vi "Convert SAP CTCL Report File to Table.vi"(0 "File Path":path=path "C:/Users/rgenaway/Documents/Singapore Schedule Control/Workcenter Reports/CTCLActivitySing.txt", 1 "Sing Time Zone":bool) -> (7 "Converted Data Table":string[][](table), 8 "last mod":u32 format="%<%I:%M:%S %p\n%m/%d/%Y>T")   [LabVIEW 2018]
uses:
  <vilib>/Utility/file.llb/Read Delimited Spreadsheet (string).vi
panel:
  out "Start Index":i32
  out "all rows":string[][](array[string])
  # "This VI is used to convert a SAP text file into a Labview Table."
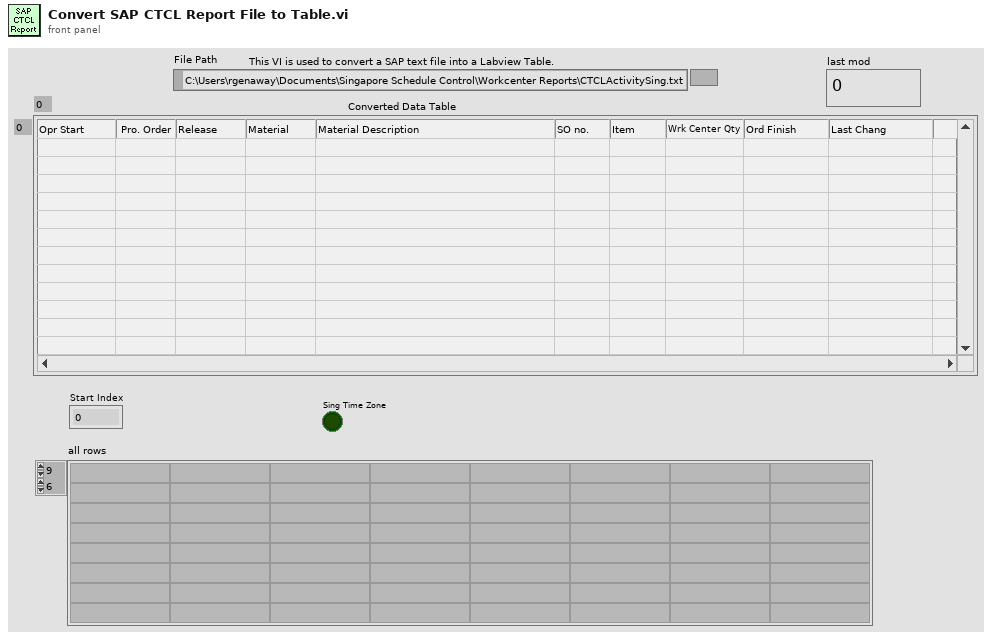
[diagram p1: front panel]
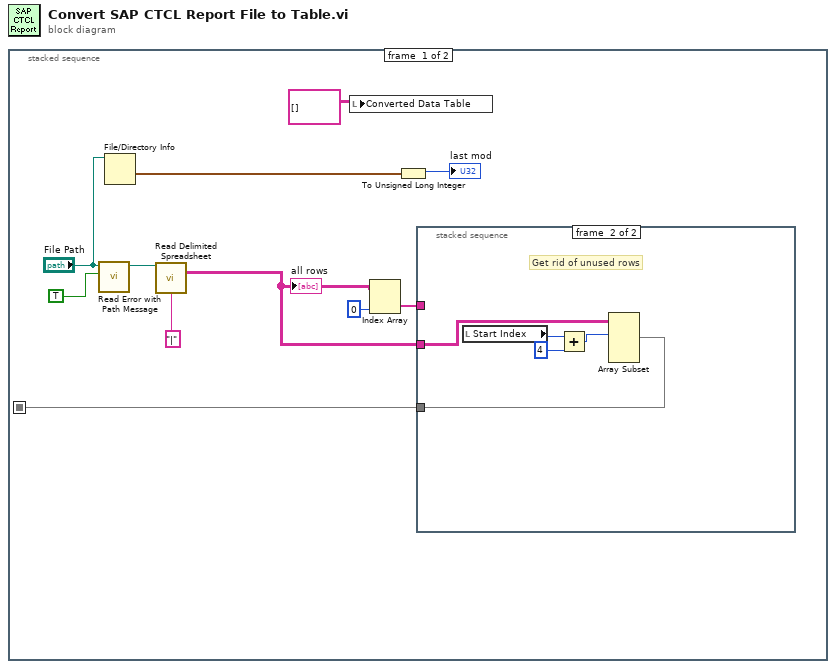
[diagram p0: block diagram]
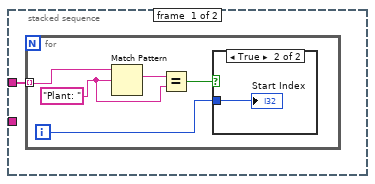
[diagram p2: hidden frame]
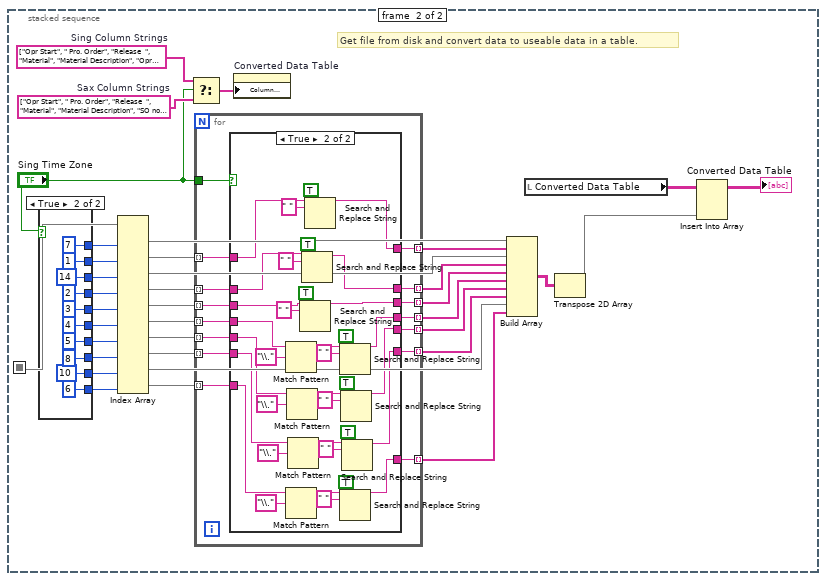
[diagram p4: hidden frame]
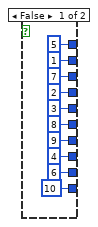
[diagram p5: hidden frame]
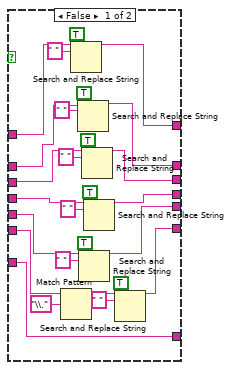
[diagram p6: hidden frame]
diagram:
  n1 = stacked-sequence {
    seq-local: [w8 _] -> [_ w46]
    frame #0 {
      n2 = call "Read Error with Path Message.vi"("quit? (T)"=TRUE, "Path"="File Path") -> ("path out"=w3:path)  [unwired: 8 in, 1 out]
      n3 = File/Directory Info(path="File Path") -> (last mod=w11:timestamp)  [unwired: 1 in, 6 out]
      n4 = call-poly <vilib>:"Read Delimited Spreadsheet.vi"("file path (dialog if empty)"=w3, "delimiter (\\t)"="|" ("delimiter (\\t)")) -> ("all rows"=w1:string[][])  [unwired: 8 in, 5 out]
      "all rows" <- w1
      n5 = local write "Converted Data Table"(string[][] [] ("Table")) -> ()
      n6 = Index Array(array=w1, index (col)=0 ("disabled index (col)")) -> (element=w5:string[])  [unwired: 1 in]
      n7 = To Unsigned Long Integer(number=w11) -> (unsigned 32bit integer=→"last mod":u32)
      n8 = stacked-sequence {
        tunnel: w5 -> [w12 _]
        tunnel: w1 -> [_ w23]
        tunnel: [_ w22] -> w8
        frame #0 {
          n9 = for {
            tunnel: w12 -> [w17] mode=indexing
            i -> [w13]
            w15 = "Plant: "
            n10 = Match Pattern(string=w17, regular expression=w15) -> (match substring=w16:string)  [unwired: 1 in, 3 out]
            n11 = Equal?(x=w16, y=w15) -> (x = y?=w14:bool)
            n12 = case shown="True" w14 {
              tunnel: w13 -> [_ w18]
              frame False {
              }
              frame True {
                "Start Index" <- w18
              }
            }
          }
        }
        frame #1 {
          # "Get rid of unused rows"
          n13 = local read "Start Index"() -> (w21:i32)
          n14 = Add(x=w21, y=4) -> (x+y=w19:i32)
          n15 = Array Subset(array=w23, index (row)=w19) -> (w22:string[][])  [unwired: 3 in]
        }
      }
    }
    frame #1 {
      w30 = string[] ["Opr Start", " Pro. Order", "Release  ", "Material", "Material Description", "Opr Qty", "Conf. Qty", "Wrk Center Qty", "Ord Finish", "Open Qty"]  # Sing Column Strings
      w29 = string[] ["Opr Start", " Pro. Order", "Release  ", "Material", "Material Description", "SO no.", "Item", "Wrk Center Qty", "Ord Finish", "Last Chang"]  # Sax Column Strings
      # "Get file from disk and convert data to useable data in a table."
      n16 = case shown="True" "Sing Time Zone" {
        tunnel: [5 ("disabled index (col)") 7 ("disabled index (col)")] -> w56
        tunnel: [1 ("index (col)") 1 ("index (col)")] -> w55
        tunnel: [7 ("index (col)") 14 ("index (col)")] -> w54
        tunnel: [2 ("index (col)") 2 ("index (col)")] -> w53
        tunnel: [3 ("index (col)") 3 ("index (col)")] -> w52
        tunnel: [8 ("index (col)") 4 ("index (col)")] -> w51
        tunnel: [9 ("index (col)") 5 ("index (col)")] -> w50
        tunnel: [4 ("index (col)") 8 ("index (col)")] -> w49
        tunnel: [6 ("index (col)") 10 ("index (col)")] -> w48
        tunnel: [10 ("index (col)") 6 ("index (col)")] -> w45
        frame False {
        }
        frame True {
        }
      }
      n17 = Index Array(array=w46, index (col) #1=w56, index (col) #2=w55, index (col) #3=w54, index (col) #4=w53, index (col) #5=w52, index (col) #6=w51, index (col) #7=w50, index (col) #8=w49, index (col) #9=w48, index (col) #10=w45) -> (element #1=w42:string[], element #2=w41:string[], element #3=w39:string[], element #4=w38:string[], element #5=w27:string[], element #6=w36:string[], element #7=w34:string[], element #8=w44:string[], element #9=w32:string[], element #10=w25:string[])  [unwired: 10 in]
      n18 = Select(t=w30, s="Sing Time Zone", f=w29) -> (s? t:f=w31:string[])
      n19 = for {
        tunnel: w44 -> [w94] mode=indexing
        tunnel: [w85] -> w43 mode=indexing
        tunnel: w41 -> [w93] mode=indexing
        tunnel: [w92] -> w40 mode=indexing
        tunnel: w38 -> [w91] mode=indexing
        tunnel: [w90] -> w37 mode=indexing
        tunnel: w36 -> [w89] mode=indexing
        tunnel: [w88] -> w35 mode=indexing
        tunnel: w34 -> [w87] mode=indexing
        tunnel: [w86] -> w33 mode=indexing
        tunnel: "Sing Time Zone" -> [w84]
        tunnel: w27 -> [w83] mode=indexing
        tunnel: [w82] -> w26 mode=indexing
        tunnel: w25 -> [w81] mode=indexing
        tunnel: [w80] -> w24 mode=indexing
        n20 = case shown="True" w84 {
          tunnel: w94 -> [w121 w137]
          tunnel: w93 -> [w109 w123]
          tunnel: [w108 w122] -> w92
          tunnel: w91 -> [w107 w127]
          tunnel: [w106 w126] -> w90
          tunnel: w89 -> [w105 w149]
          tunnel: [w104 w148] -> w88
          tunnel: w87 -> [w103 w143]
          tunnel: [w102 w142] -> w86
          tunnel: [w100 w136] -> w85
          tunnel: w83 -> [w97 w155]
          tunnel: [w96 w154] -> w82
          tunnel: w81 -> [w95 w131]
          tunnel: [w95 w130] -> w80
          frame False {
            n21 = Match Pattern(string=w121, regular expression="\\.") -> (before substring=w101:string)  [unwired: 1 in, 3 out]
            n22 = Search and Replace String(replace all?=TRUE ("replace all? (F)"), input string=w109, search string=" ") -> (result string=w108:string)  [unwired: 5 in, 3 out]
            n23 = Search and Replace String(replace all?=TRUE ("replace all? (F)"), input string=w107, search string=" ") -> (result string=w106:string)  [unwired: 5 in, 3 out]
            n24 = Search and Replace String(replace all?=TRUE ("replace all? (F)"), input string=w103, search string=" ") -> (result string=w102:string)  [unwired: 5 in, 3 out]
            n25 = Search and Replace String(replace all?=TRUE ("replace all? (F)"), input string=w97, search string=" ") -> (result string=w96:string)  [unwired: 5 in, 3 out]
            n26 = Search and Replace String(replace all?=TRUE ("replace all? (F)"), input string=w105, search string=" ") -> (result string=w104:string)  [unwired: 5 in, 3 out]
            n27 = Search and Replace String(replace all?=TRUE ("replace all? (F)"), input string=w101, search string=" ") -> (result string=w100:string)  [unwired: 5 in, 3 out]
          }
          frame True {
            n28 = Match Pattern(string=w149, regular expression="\\.") -> (before substring=w150:string)  [unwired: 1 in, 3 out]
            n29 = Match Pattern(string=w131, regular expression="\\.") -> (before substring=w132:string)  [unwired: 1 in, 3 out]
            n30 = Match Pattern(string=w143, regular expression="\\.") -> (before substring=w144:string)  [unwired: 1 in, 3 out]
            n31 = Match Pattern(string=w137, regular expression="\\.") -> (before substring=w138:string)  [unwired: 1 in, 3 out]
            n32 = Search and Replace String(replace all?=TRUE ("replace all? (F)"), input string=w155, search string=" ") -> (result string=w154:string)  [unwired: 5 in, 3 out]
            n33 = Search and Replace String(replace all?=TRUE ("replace all? (F)"), input string=w127, search string=" ") -> (result string=w126:string)  [unwired: 5 in, 3 out]
            n34 = Search and Replace String(replace all?=TRUE ("replace all? (F)"), input string=w123, search string=" ") -> (result string=w122:string)  [unwired: 5 in, 3 out]
            n35 = Search and Replace String(replace all?=TRUE ("replace all? (F)"), input string=w150, search string=" ") -> (result string=w148:string)  [unwired: 5 in, 3 out]
            n36 = Search and Replace String(replace all?=TRUE ("replace all? (F)"), input string=w132, search string=" ") -> (result string=w130:string)  [unwired: 5 in, 3 out]
            n37 = Search and Replace String(replace all?=TRUE ("replace all? (F)"), input string=w144, search string=" ") -> (result string=w142:string)  [unwired: 5 in, 3 out]
            n38 = Search and Replace String(replace all?=TRUE ("replace all? (F)"), input string=w138, search string=" ") -> (result string=w136:string)  [unwired: 5 in, 3 out]
          }
        }
      }
      n39 = property on="Converted Data Table" class="Tbl (strict)"("Column Headers[]"=w31) -> ()  [unwired: 2 in, 2 out]
      n40 = Build Array(w42, w40, w39, w37, w26, w35, w33, w43, w32, w24) -> (w57:string[][])
      n41 = local read "Converted Data Table"() -> (w59:string[][])
      n42 = Transpose 2D Array(2D array=w57) -> (transposed array=w47:string[][])
      n43 = Insert Into Array(array=w59, new element=w47) -> (→"Converted Data Table":string[][])  [unwired: 2 in]
    }
  }
